vi "FirstPrac.vi"() -> ()   [LabVIEW 2018]
panel:
  out "Waveform Graph":cluster{dbl, dbl, dbl[]}(graph)
  in  "Stop":bool
  out "Waveform Chart":dbl(graph)
  out "String controller":string
  in  "String":string
  out "C * ( A + B )":dbl
  in  "Value C":dbl
  out "Counter":dbl
  in  "stop":bool
  out "A + B":dbl
  in  "Value B":dbl
  in  "Value A":dbl
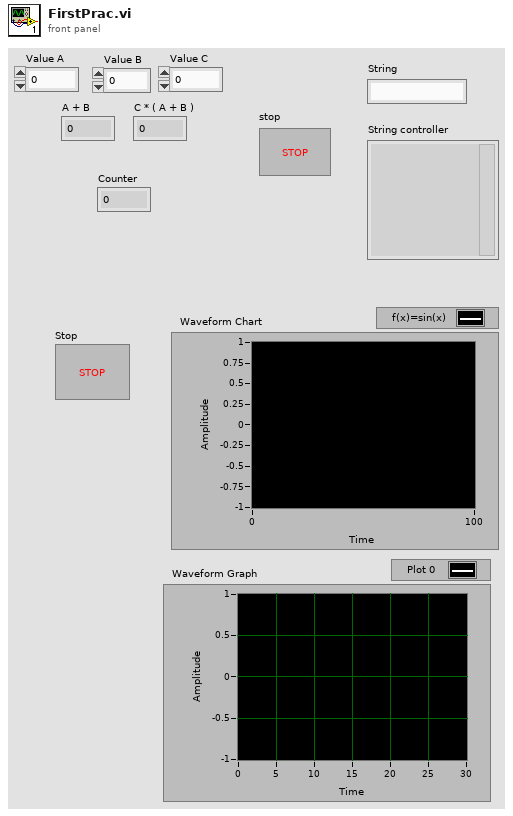
[diagram p1: front panel]
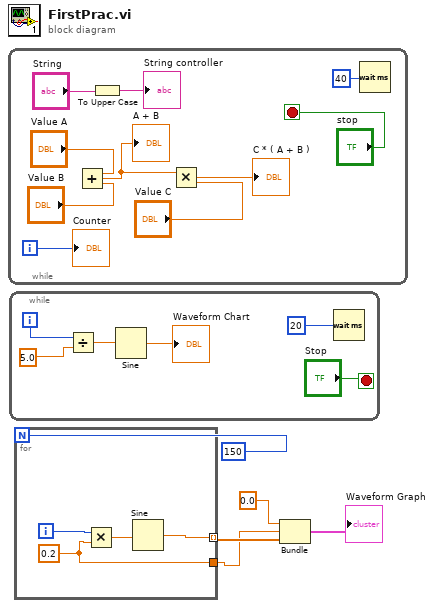
[diagram p0: block diagram]
diagram:
  n1 = while {
    i -> [w12]
    stop <- "stop" stop-if-true
    n2 = Add(x="Value A", y="Value B") -> (x+y=w11:dbl)
    "A + B" <- w11
    n3 = To Upper Case(1:"String") -> (0:→"String controller":string)
    n4 = Multiply(x=w11, y="Value C") -> (x*y=→"C * ( A + B )":dbl)
    n5 = Wait (ms)(milliseconds to wait=u32 40) -> ()  [unwired: 1 out]
    "Counter" <- w12
  }
  n6 = while {
    i -> [w17]
    stop <- "Stop" stop-if-true
    n7 = Divide(x=w17, y=5.0) -> (x/y=w19:dbl)
    n8 = Sine(x=w19) -> (sin(x)=→"Waveform Chart":dbl)
    n9 = Wait (ms)(milliseconds to wait=20) -> ()  [unwired: 1 out]
  }
  n10 = for {
    N: 150 -> [_]
    tunnel: [w25] -> w3 mode=indexing
    tunnel: [w22] -> w1
    i -> [w23]
    w22 = 0.2
    n11 = Multiply(x=w23, y=w22) -> (x*y=w24:dbl)
    n12 = Sine(x=w24) -> (sin(x)=w25:dbl)
  }
  n13 = Bundle(0.0, w1, w3) -> (→"Waveform Graph":cluster{dbl, dbl, dbl[]})  [unwired: 1 in]
